vi "ClimberCalc.vi"(0 "Climber_Commands":T3, 1 "Climber Inputs":T1) -> (7 "Climber_Outputs":T2)   [LabVIEW 2012]
uses:
  Climber_Commands.ctl
  Climber_Outputs.ctl
  climber_sensor_readings.ctl
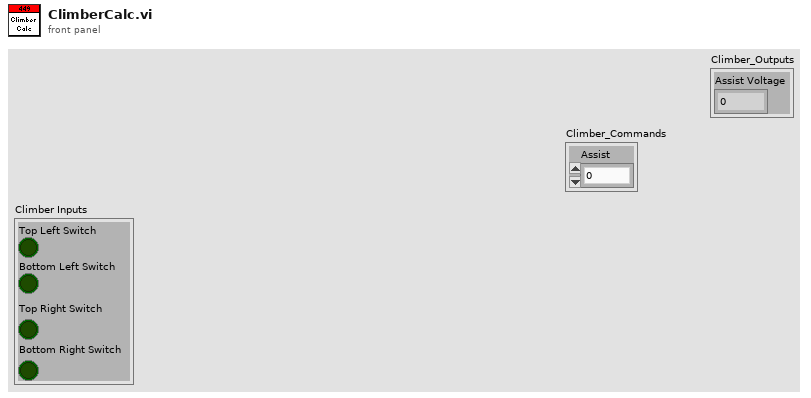
[diagram p1: front panel]
types:
  T1 = typedef "climber_sensor_readings.ctl" = cluster{"Top Left Switch":bool, "Bottom Left Switch":bool, "Top Right Switch":bool, "Bottom Right Switch":bool}
  T2 = typedef "Climber_Outputs.ctl" = cluster{"Assist Voltage":dbl}
  T3 = typedef "Climber_Commands.ctl" = cluster{"Assist":dbl}
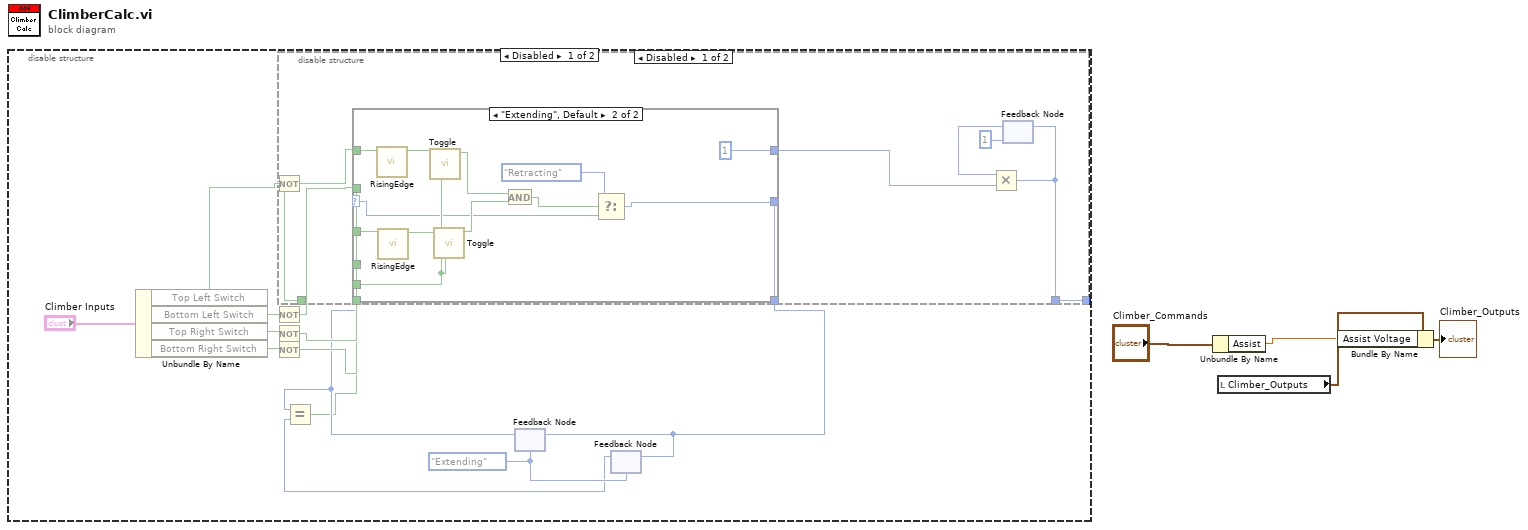
[diagram p0: block diagram]
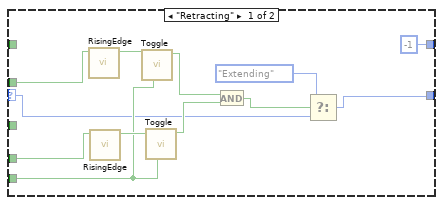
[diagram p2: hidden frame]
diagram:
  n1 = disable-structure shown="Disabled" {
    disable-tunnel: [w18 _] -> _
    frame Disabled {
      w8 = enum16{"Extending", "Retracting"}."Extending"
      n2 = Unbundle By Name("Climber Inputs") -> ("Top Left Switch"=w13:bool, "Bottom Left Switch"=w14:bool, "Top Right Switch"=w15:bool, "Bottom Right Switch"=w16:bool)
      n3 = Not(x=w14) -> (.not. x?=w12:bool)
      n4 = Not(x=w15) -> (.not. x?=w11:bool)
      n5 = Not(x=w16) -> (.not. x?=w10:bool)
      n6 = feedback #1(w8) -> (w6:enum16{"Extending", "Retracting"})
      n7 = feedback #2(w8) -> (w7:enum16{"Extending", "Retracting"})
      n8 = Equal?(x=w6, y=w7) -> (x = y?=w5:bool)
      n9 = disable-structure shown="Disabled" {
        disable-tunnel: [w28 _] -> w18
        disable-tunnel: w13 -> [w27 _]
        disable-tunnel: w12 -> [w25 _]
        disable-tunnel: w11 -> [w24 _]
        disable-tunnel: w10 -> [w23 _]
        disable-tunnel: [w22 _] -> w9
        disable-tunnel: w6 -> [w21 _]
        disable-tunnel: w5 -> [w20 _]
        frame Disabled {
          n10 = Not(x=w27) -> (.not. x?=w26:bool)
          n11 = case shown="\"Extending\", Default" w21 {
            selector: w21 -> [w32 w46]
            tunnel: [w31 w45] -> w22
            tunnel: w26 -> [_ w54]
            tunnel: w25 -> [w35 _]
            tunnel: w24 -> [_ w53]
            tunnel: w23 -> [w34 _]
            tunnel: w20 -> [w33 w50]
            tunnel: [-1 1] -> w19
            frame "Retracting" {
              n12 = call "RisingEdge.vi"("BooleanIn"=w35) -> ("BooleanOut"=w41:bool)  [unwired: 10 in]
              n13 = call "RisingEdge.vi"("BooleanIn"=w34) -> ("BooleanOut"=w40:bool)  [unwired: 10 in]
              n14 = call "Toggle.vi"("Reset"=w33, "Toggle"=w41) -> ("BoolOut"=w39:bool)  [unwired: 9 in]
              n15 = call "Toggle.vi"("Reset"=w33, "Toggle"=w40) -> ("BoolOut"=w38:bool)  [unwired: 9 in]
              n16 = And(x=w39, y=w38) -> (x .and. y?=w37:bool)
              n17 = Select(t=enum16{"Extending", "Retracting"}."Extending", s=w37, f=w32) -> (s? t:f=w31:enum16{"Extending", "Retracting"})
            }
            frame "Extending", Default {
              n18 = call "RisingEdge.vi"("BooleanIn"=w54) -> ("BooleanOut"=w52:bool)  [unwired: 10 in]
              n19 = call "RisingEdge.vi"("BooleanIn"=w53) -> ("BooleanOut"=w51:bool)  [unwired: 10 in]
              n20 = call "Toggle.vi"("Reset"=w50, "Toggle"=w52) -> ("BoolOut"=w49:bool)  [unwired: 9 in]
              n21 = call "Toggle.vi"("Reset"=w50, "Toggle"=w51) -> ("BoolOut"=w48:bool)  [unwired: 9 in]
              n22 = And(x=w49, y=w48) -> (x .and. y?=w47:bool)
              n23 = Select(t=enum16{"Extending", "Retracting"}."Retracting", s=w47, f=w46) -> (s? t:f=w45:enum16{"Extending", "Retracting"})
            }
          }
          n24 = feedback #3(i16 1 ("Arm Direction")) -> (w29:i16)
          n25 = Multiply(x=w29, y=w19) -> (x*y=w28:i32)
          n26 = feedback-in #3(w28) -> ()
        }
        frame Enabled {
        }
      }
      n27 = feedback-in #1(w9) -> ()
      n28 = feedback-in #2(w9) -> ()
    }
    frame Enabled {
    }
  }
  n29 = Unbundle By Name("Climber_Commands") -> ("Assist"=w1:dbl)
  n30 = local read "Climber_Outputs"() -> (w4:T2)
  n31 = Bundle By Name(cluster=w4, "Assist Voltage"=w1) -> (→"Climber_Outputs":T2)
